vi "SLL DE AO Circular Buffer.vi"(6 "Pointers":T3=enum."Pointer 4", 7 "Options":T4=enum."Write N", 8 "error in (no error)":errorcluster, 11 "AO value Array":dbl[][](array[numeric])) -> (0 "error Out":errorcluster, 1 "Data Overflow?":T2, 2 "Output points":sgl[](array[numeric]), 3 "Output Data":sgl[][](array[numeric]))   [LabVIEW 2013]
doc: "This vi acts as a circular buffer for Analog input channel data storage. \nOutput Array- Column coresponds to single channel data.\nSingle Point data of all channels will avilable, When 'Data Point' case will executes.\nYou can get continous data in two mode 'Read Pointer 1' and 'Read Pointer 2'.\nInitializing Pointer is recommeded to avoid overflow\n\nCreated by Yogesh Redemptor, \nCopyright © 2009, Soliton Technologies.\nAll rights reserved."
uses:
  Controls/SLL DE AO Circular Buffer Options.ctl
  Controls/SLL DE Circular Buffer Pointers List.ctl
  Controls/SLL DE Circular Buffer Overflow Info.ctl
  Controls/SLL DE List of Analog Outputs.ctl
  Controls/SLL DE DAQ Parameters LV2Global Options.ctl
panel:
  in  "AO Channel Name Array":T1[](array[typedef])
  in  "AO value":dbl[](array[numeric])
  in  "AO Channel Name":T1
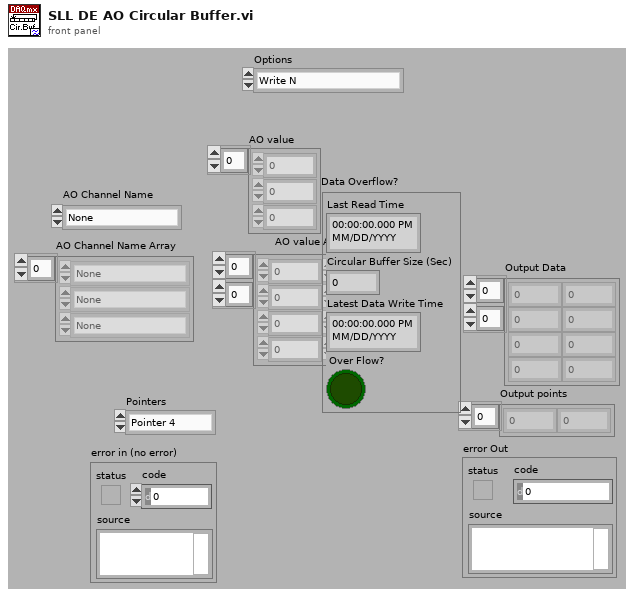
[diagram p1: front panel]
types:
  T1 = typedef "SLL DE List of Analog Outputs.ctl" = enum16{"None"}
  T2 = typedef "SLL DE Circular Buffer Overflow Info.ctl" = cluster{"Last Read Time":timestamp, "Circular Buffer Size (Sec)":dbl, "Latest Data Write Time":timestamp, "Over Flow?":bool}
  T3 = typedef "SLL DE Circular Buffer Pointers List.ctl" = enum16{"Graph Pointer", "File Log Pointer", "Pointer 3", "Pointer 4"}
  T4 = typedef "SLL DE AO Circular Buffer Options.ctl" = enum16{"Initialize", "Write 1", "Write N", "Read 1", "Read N", "Clear Data"}
  T5 = typedef "SLL DE DAQ Parameters LV2Global Options.ctl" = enum16{"Read", "Write"}
  T6 = cluster{"Buffer Length":i32, "Write Pointer":i32, "Write Time":timestamp, "AI Sampling Rate (Samples/Sec)":i32, "# Samples to write":i32}
  T7 = cluster{"Read Pointer X Pointer":i32, "Pointer X Overflow?":bool, "Read Pointer X Time":timestamp}
  T8 = typedef "SLL DE DAQ Engine Parameters.ctl" = cluster{"Enable Engines":cluster{"AI Enable":bool, "AO Enable":bool, "DI Enable":bool, "DO Enable":bool}, "DAQ Control Type":cluster{"Analog Input":enum16{"Finite", "Continuous", "Driver"}, "Analog Output":enum16{"Finite", "Continuous", "Driver"}, "Digital Input":enum16{"Finite", "Continuous", "Driver"}, "Digital Output":enum16{"Finite", "Continuous", "Driver"}}, "DAQ Parameters":cluster{"AI Sampling Rate (Samples/Sec)":dbl, "MvgAVG Window Size (# of Points)":i32, "Enable Filter":bool, "Enable MvgAVG":bool, "Circular Buffer Size (Sec)":dbl, "AO Sampling Rate (Samples/Sec)":dbl, "Graph Update Rate (Samples/Sec)":dbl, "File Logging Rate (Samples/Sec)":i32}, "AO Safe Values":cluster{"Analog Outputs Name":T1, "Analog Outputs Safe Value":dbl}[], "DO Safe Values":cluster{"Digital Outputs Name":T9, "Digital Outputs Safe Value":bool}[], "DO Interconnected Lines":cluster{"First DO Line":string, "Second DO Line":string}[], "AI Channels Unit":cluster{"Channel Name":T10, "Channel Type":T11}[], "Units Information":cluster{"Channel Type":T11, "Unit Text":string, "Maximum":dbl, "Minmum":dbl, "Increments":dbl}[]}
  T9 = typedef "SLL DE List of Digital Outputs.ctl" = enum16{"STATION1_START TEST", "STATION1_STOP TEST", "STATION1_LIGHT1", "STATION1_LIGHT2", "STATION1_LIGHT3", "STATION2_START TEST", "STATION2_STOP TEST", "STATION2_LIGHT1", "STATION2_LIGHT2", "STATION2_LIGHT3", "STATION3_START TEST", "STATION3_STOP TEST", "STATION3_LIGHT1", "STATION3_LIGHT2", "STATION3_LIGHT3", "STATION4_START TEST", "STATION4_STOP TEST", "STATION4_LIGHT1", "STATION4_LIGHT2", "STATION4_LIGHT3"}
  T10 = typedef "SLL DE List of Analog Inputs.ctl" = enum16{"None"}
  T11 = typedef "SLL DE List of AI Channel Type.ctl" = enum16{"Pressure", "Flow", "Temperature", "Time Scale", "Voltage", "Current", "Frequency", "Sound", "Speed", "Torque", "Distance", "Channel Type 1", "Channel Type 2", "Channel Type 3"}
  T12 = cluster{"Read Pointer X Pointer":i32, "Pointer X Overflow?":bool, "Read Pointer X Time":timestamp}[]
  T13 = cluster{"Read Pointer X Time":timestamp, "Circular Buffer Size (Sec)":dbl, "Write Time":timestamp, bool}
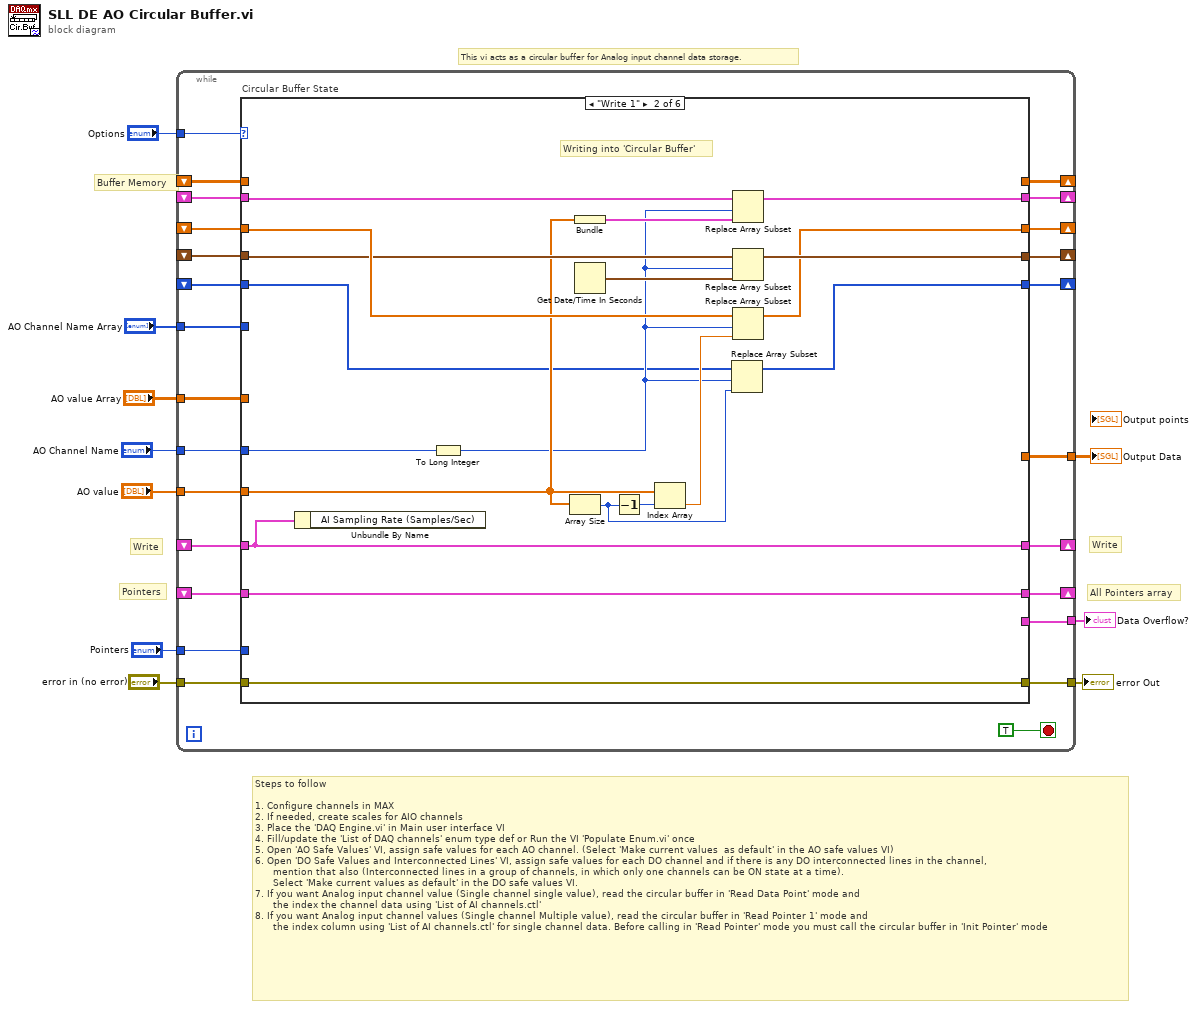
[diagram p0: block diagram]
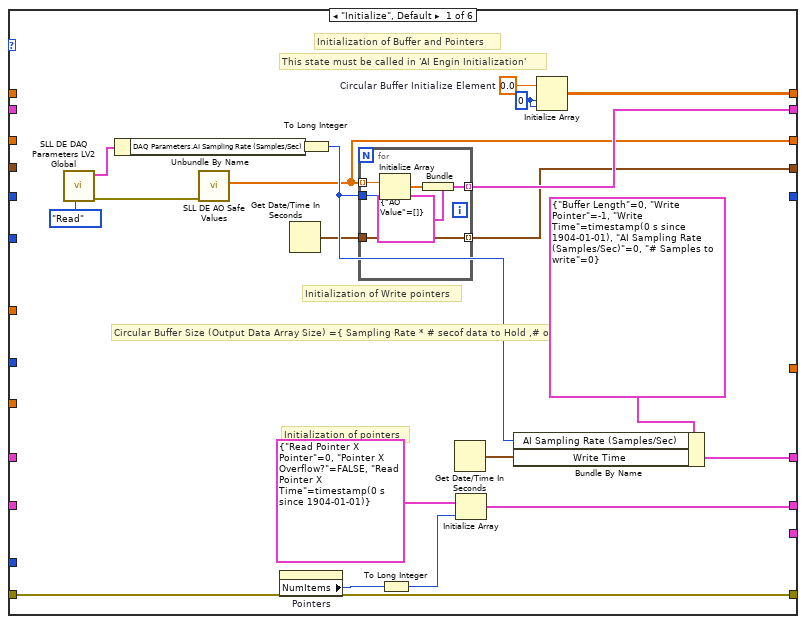
[diagram p2: hidden frame]
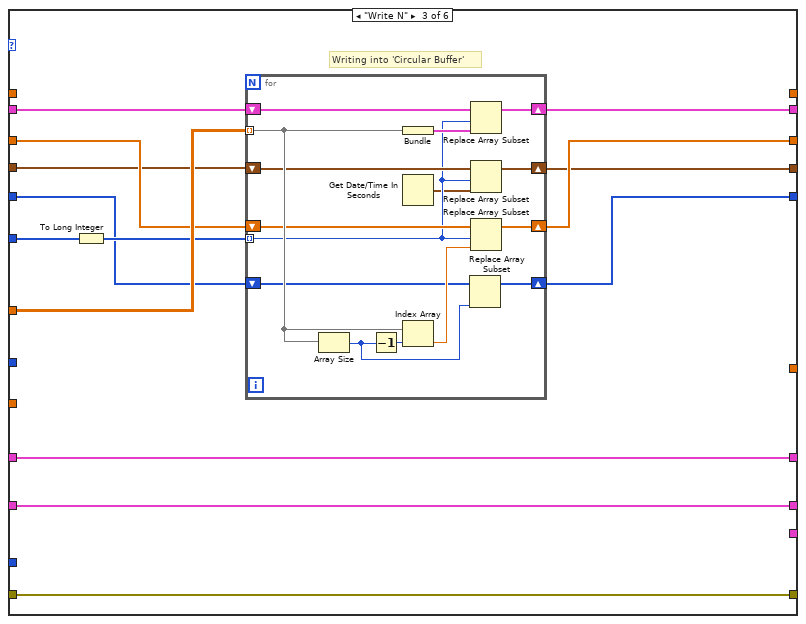
[diagram p3: hidden frame]
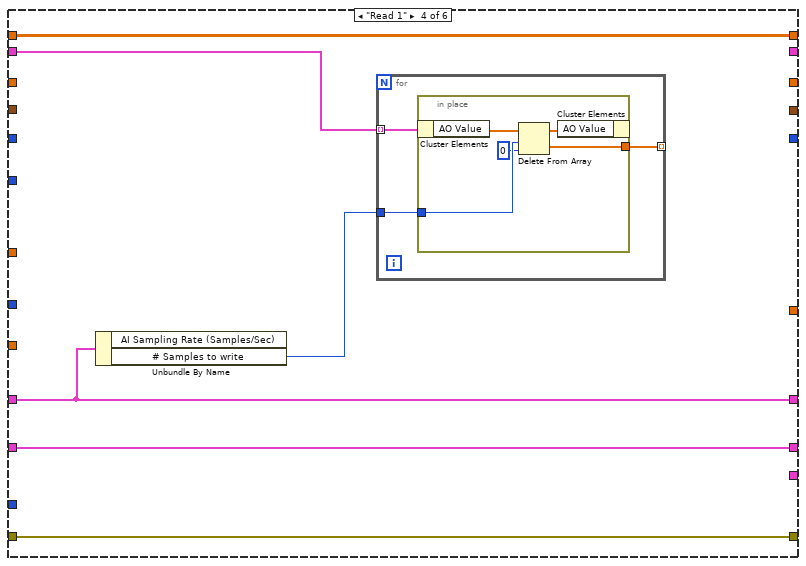
[diagram p4: hidden frame]
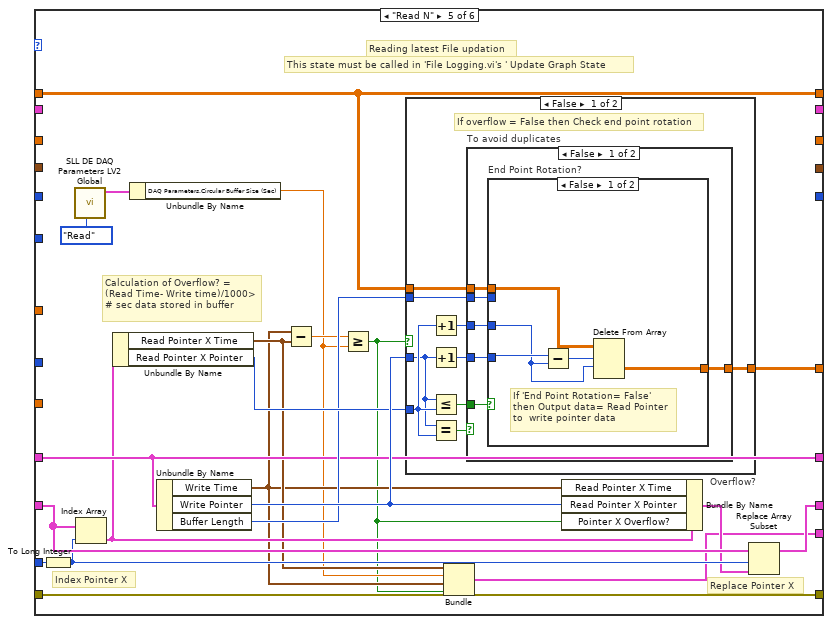
[diagram p5: hidden frame]
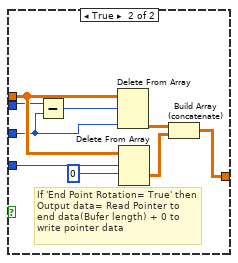
[diagram p6: hidden frame]
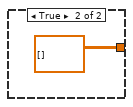
[diagram p7: hidden frame]
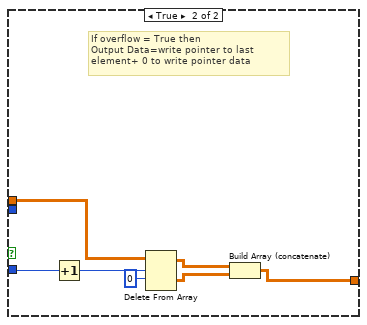
[diagram p8: hidden frame]
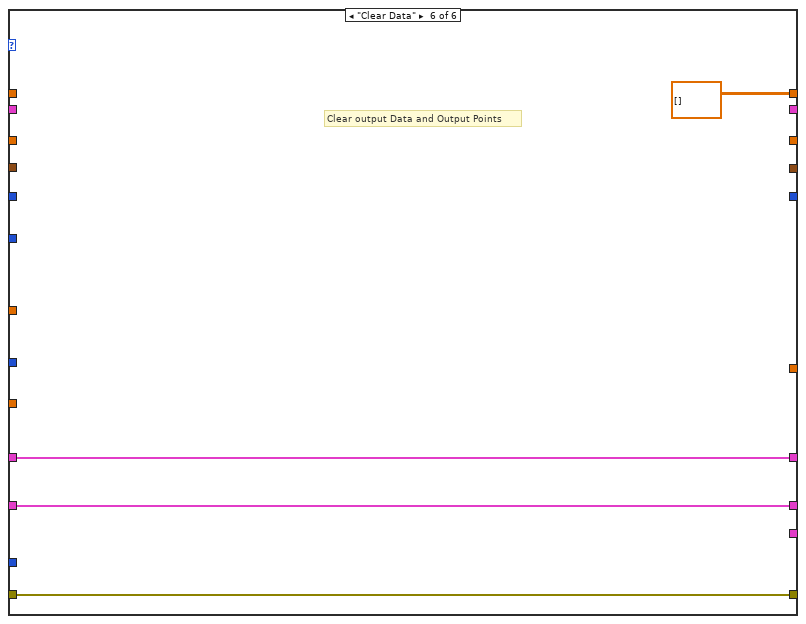
[diagram p9: hidden frame]
diagram:
  # "Steps to follow\n\n1.\tConfigure channels in MAX\n2.\tIf needed, create scales for AIO channels\n3.\tPlace the 'DAQ Engine.vi' in Main user interface VI\n4.\tFill/update the 'List of DAQ channels' enum type def or Run the VI 'Populate Enum.vi' once\n5.\tOpen 'AO Safe Values' VI, assign safe values for each AO channel. (Select 'Make current values  as default' in the AO safe values VI)\n6.\tOpen 'DO Safe Values and Interconnected Lines' VI, assign safe values for each DO channel and if there is any DO interconnected lines in the channel,\n      mention that also (Interconnected lines in a group of channels, in which only one channels can be ON state at a time). \n      Select 'Make current values as default' in the DO safe values VI.\n7.\tIf you want Analog input channel value (Single channel single value), read the circular buffer in 'Read Data Point' mode and \n      the index the channel data using 'List of AI channels.ctl' \n8.\tIf you want Analog input channel values (Single channel Multiple value), read the circular buffer in 'Read Pointer 1' mode and \n      the index column using 'List of AI channels.ctl' for single channel data. Before calling in 'Read Pointer' mode you must call the circular buffer in 'Init Pointer' mode"
  # "Buffer Memory"
  # "Write"
  # "Write"
  # "Pointers"
  # "All Pointers array"
  # "This vi acts as a circular buffer for Analog input channel data storage."
  n1 = while {
    tunnel: "Options" -> [w35]
    shift-right: [w33] -> _
    shift-left: _ -> [w31]
    shift-right: [w32] -> _
    shift-left: _ -> [w30]
    tunnel: "AO value Array" -> [w29]
    shift-right: [w28] -> _
    shift-left: _ -> [w27]
    tunnel: [w26] -> w9
    tunnel: "error in (no error)" -> [w25]
    tunnel: [w24] -> w7
    tunnel: "Pointers" -> [w23]
    tunnel: [w22] -> w4
    shift-right: [w21] -> _
    shift-left: _ -> [w20]
    tunnel: "AO Channel Name" -> [w19]
    tunnel: "AO value" -> [w18]
    tunnel: "AO Channel Name Array" -> [w17]
    shift-right: [w16] -> _
    shift-left: _ -> [w15]
    shift-right: [w14] -> _
    shift-left: _ -> [w13]
    shift-right: [w12] -> _
    shift-left: _ -> [w11]
    stop <- TRUE stop-if-true
    n2 = case "Circular Buffer State" shown="\"Write 1\"" w35 {
      tunnel: [w55 _ _ w114 w144 sgl[][] []] -> w33
      tunnel: [w51 w76 w94 w115 w133 w185] -> w32
      tunnel: w31 -> [_ _ _ w114 w144 _]
      tunnel: w30 -> [_ w76 w94 w115 w136 w185]
      tunnel: w29 -> [_ _ w92 _ _ _]
      tunnel: [w52 w75 w83 w112 w139 w184] -> w28
      tunnel: w27 -> [_ w75 w83 w112 w139 w184]
      tunnel: [_ _ _ _ w143 _] -> w26
      tunnel: w25 -> [w47 w80 w93 w113 w138 w182]
      tunnel: [w47 w80 w93 w113 w138 w182] -> w24
      tunnel: w23 -> [_ _ _ _ w137 _]
      tunnel: [_ _ _ _ w124 _] -> w22
      tunnel: [w41 w72 w88 _ _ _] -> w21
      tunnel: w20 -> [_ w79 w91 w111 _ _]
      tunnel: w19 -> [_ w67 _ _ _ _]
      tunnel: w18 -> [_ w66 _ _ _ _]
      tunnel: w17 -> [_ _ w90 _ _ _]
      tunnel: [w38 w73 w87 _ _ _] -> w16
      tunnel: w15 -> [_ w78 w86 _ _ _]
      tunnel: [w36 w74 w84 _ _ _] -> w14
      tunnel: w13 -> [_ w77 w85 _ _ _]
      tunnel: [_ w63 w81 _ _ _] -> w12
      tunnel: w11 -> [_ w62 w82 _ _ _]
      frame "Initialize", Default {
        w54 = sgl 0.0  # Circular Buffer Initialize Element
        w43 = 0 ("dimension size")
        # "Initialization of pointers"
        # "Initialization of Write pointers"
        # "This state must be called in 'AI Engin Initialization'"
        # "Initialization of Buffer and Pointers"
        # "Circular Buffer Size (Output Data Array Size) ={ Sampling Rate * # secof data to Hold ,# of AI Channels}"
        n3 = call "SLL DE DAQ Parameters LV2 Global.vi"("Option"=SLL_DE_DAQ_Parameters_LV2Global_Options."Read") -> ("Error out"=w40:errorcluster, "Global Info"=w48:T8)  [unwired: 9 in]
        n4 = Unbundle By Name(w48) -> ("DAQ Parameters.AI Sampling Rate (Samples/Sec)"=w42:dbl)
        n5 = call "SLL DE AO Safe Values.vi"("error in (no error)"=w40) -> ("AO Safe Values"=w38:dbl[])  [unwired: 8 in, 2 out]
        n6 = property on="Pointers" class="Enum (strict)"() -> ("NumItems"=w46:u32)  [unwired: 2 in, 2 out]
        n7 = Get Date/Time In Seconds() -> (seconds since 1Jan1904=w37:timestamp)
        n8 = To Long Integer(number=w42) -> (32bit integer=w39:i32)
        n9 = for {
          tunnel: w38 -> [w61] mode=indexing
          tunnel: w39 -> [w60]
          tunnel: [w58] -> w41 mode=indexing
          tunnel: w37 -> [w57]
          tunnel: [w57] -> w36 mode=indexing
          n10 = Initialize Array(w61, w60) -> (w59:dbl[])
          n11 = Bundle(cluster=cluster{"AO Value":dbl[]} {"AO Value"=[]}, "AO Value"=w59) -> (w58:cluster{"AO Value":dbl[]})
        }
        n12 = To Long Integer(number=w46) -> (32bit integer=w45:i32)
        n13 = Get Date/Time In Seconds() -> (seconds since 1Jan1904=w44:timestamp)
        n14 = Initialize Array(T7 {"Read Pointer X Pointer"=0, "Pointer X Overflow?"=FALSE, "Read Pointer X Time"=timestamp(0 s since 1904-01-01)} ("Graph"), w45) -> (w51:T12)
        n15 = Bundle By Name(cluster=T6 {"Buffer Length"=0, "Write Pointer"=-1, "Write Time"=timestamp(0 s since 1904-01-01), "AI Sampling Rate (Samples/Sec)"=0, "# Samples to write"=0} ("Cluster"), "AI Sampling Rate (Samples/Sec)"=w39, "Write Time"=w44) -> (w52:T6)
        n16 = Initialize Array(w54, w43, w43) -> (w55:sgl[][])
      }
      frame "Write 1" {
        # "Writing into 'Circular Buffer'"
        n17 = Unbundle By Name(w75) -> ()  [unwired: 1 out]
        n18 = To Long Integer(number=w67) -> (32bit integer=w64:i32)
        n19 = Array Size(array=w66) -> (size(s)=w65:i32)
        n20 = Bundle("AO value"=w66) -> (w71:cluster{"AO value":dbl[]})  [unwired: 1 in]
        n21 = Get Date/Time In Seconds() -> (seconds since 1Jan1904=w68:timestamp)
        n22 = Decrement(x=w65) -> (x-1=w70:i32)
        n23 = Index Array(array=w66, index=w70) -> (element=w69:dbl)
        n24 = Replace Array Subset(array=w62, new element=w65, index=w64) -> (w63:i32[])
        n25 = Replace Array Subset(array=w79, new element=w71, index=w64) -> (w72:cluster{"AO Value":dbl[]}[])
        n26 = Replace Array Subset(array=w77, new element=w68, index=w64) -> (w74:timestamp[])
        n27 = Replace Array Subset(array=w78, new element=w69, index=w64) -> (w73:dbl[])
      }
      frame "Write N" {
        # "Writing into 'Circular Buffer'"
        n28 = To Long Integer(number=w90) -> (32bit integer=w89:i32[])
        n29 = for {
          tunnel: w92 -> [w105] mode=indexing
          shift-right: [w108] -> w88
          shift-left: w91 -> [w109]
          tunnel: w89 -> [w99] mode=indexing
          shift-right: [w103] -> w87
          shift-left: w86 -> [w102]
          shift-right: [w100] -> w84
          shift-left: w85 -> [w101]
          shift-right: [w96] -> w81
          shift-left: w82 -> [w95]
          n30 = Array Size(array=w105) -> (size(s)=w97:i32)
          n31 = Decrement(x=w97) -> (x-1=w106:i32)
          n32 = Bundle("AO value Array"=w105) -> (w107:cluster{"AO value Array":dbl[]})  [unwired: 1 in]
          n33 = Get Date/Time In Seconds() -> (seconds since 1Jan1904=w98:timestamp)
          n34 = Index Array(array=w105, index=w106) -> (element=w104:dbl)
          n35 = Replace Array Subset(array=w95, new element=w97) -> (w96:i32[])  [unwired: 1 in]
          n36 = Replace Array Subset(array=w109, new element=w107, index=w99) -> (w108:cluster{"AO Value":dbl[]}[])
          n37 = Replace Array Subset(array=w101, new element=w98, index=w99) -> (w100:timestamp[])
          n38 = Replace Array Subset(array=w102, new element=w104, index=w99) -> (w103:dbl[])
        }
      }
      frame "Read 1" {
        n39 = Unbundle By Name(w112) -> ("# Samples to write"=w110:i32)  [unwired: 1 out]
        n40 = for {
          tunnel: w111 -> [w118] mode=indexing
          tunnel: w110 -> [w117]
          tunnel: [w116] -> _ mode=indexing
          n41 = in-place {
            in-place-border: w117 -> [w120]
            in-place-border: [w121] -> w116
            n42 = in-place-cluster #1(w118) -> ("AO Value"=w123:dbl[])
            n43 = Delete From Array(array=w123, length=w120, index=0) -> (deleted portion=w121:dbl[], array with subset deleted=w122:dbl[])
            n44 = in-place-cluster #1("AO Value"=w122) -> ()  [unwired: 1 out]
          }
        }
      }
      frame "Read N" {
        # "Replace Pointer X"
        # "Index Pointer X"
        # "Calculation of Overflow? = \n(Read Time- Write time)/1000> # sec data stored in buffer"
        # "Reading latest File updation"
        # "This state must be called in 'File Logging.vi's ' Update Graph State"
        n45 = To Long Integer(number=w137) -> (32bit integer=w135:i32)
        n46 = call "SLL DE DAQ Parameters LV2 Global.vi"("Option"=SLL_DE_DAQ_Parameters_LV2Global_Options."Read") -> ("Global Info"=w131:T8)  [unwired: 9 in, 1 out]
        n47 = Index Array(array=w136, index=w135) -> (element=w132:T7)
        n48 = Unbundle By Name(w132) -> ("Read Pointer X Time"=w128:timestamp, "Read Pointer X Pointer"=w141:i32)
        n49 = Unbundle By Name(w131) -> ("DAQ Parameters.Circular Buffer Size (Sec)"=w126:dbl)
        n50 = Unbundle By Name(w139) -> ("Write Time"=w127:timestamp, "Write Pointer"=w142:i32, "Buffer Length"=w140:i32)
        n51 = Subtract(x=w127, y=w128) -> (x-y=w129:dbl)
        n52 = Greater Or Equal?(x=w129, y=w126) -> (x >= y?=w125:bool)
        n53 = case "Overflow?" shown="False" w125 {
          tunnel: w144 -> [w152 w179]
          tunnel: [w151 w177] -> w143
          tunnel: w142 -> [w147 w181]
          tunnel: w141 -> [w148 _]
          tunnel: w140 -> [w150 _]
          frame False {
            # "If overflow = False then Check end point rotation"
            n54 = Increment(x=w148) -> (x+1=w145:i32)
            n55 = Increment(x=w147) -> (x+1=w146:i32)
            n56 = Less Or Equal?(x=w147, y=w148) -> (x <= y?=w153:bool)
            n57 = Equal?(x=w147, y=w148) -> (x = y?=w149:bool)
            n58 = case "To avoid duplicates" shown="False" w149 {
              tunnel: w153 -> [w159 _]
              tunnel: w152 -> [w158 _]
              tunnel: [w157 sgl[][] []] -> w151
              tunnel: w150 -> [w156 _]
              tunnel: w145 -> [w155 _]
              tunnel: w146 -> [w154 _]
              frame False {
                n59 = case "End Point Rotation?" shown="False" w159 {
                  tunnel: w158 -> [w164 w173]
                  tunnel: [w163 w170] -> w157
                  tunnel: w155 -> [w160 w167]
                  tunnel: w154 -> [w162 w166]
                  tunnel: w156 -> [_ w169]
                  frame False {
                    # "If 'End Point Rotation= False' then Output data= Read Pointer to  write pointer data"
                    n60 = Subtract(x=w162, y=w160) -> (x-y=w161:i32)
                    n61 = Delete From Array(array=w164, length=w161, index (row)=w160) -> (deleted portion=w163:sgl[][])  [unwired: 1 in, 1 out]
                  }
                  frame True {
                    # "If 'End Point Rotation= True' then Output data= Read Pointer to end data(Bufer length) + 0 to write pointer data"
                    n62 = Subtract(x=w169, y=w167) -> (x-y=w168:i32)
                    n63 = Delete From Array(array=w173, length=w168, index (row)=w167) -> (deleted portion=w172:sgl[][])  [unwired: 1 in, 1 out]
                    n64 = Delete From Array(array=w173, length=w166, index (row)=0) -> (deleted portion=w171:sgl[][])  [unwired: 1 in, 1 out]
                    n65 = Build Array (concatenate)(w172, w171) -> (w170:sgl[][])
                  }
                }
              }
              frame True {
              }
            }
          }
          frame True {
            # "If overflow = True then\nOutput Data=write pointer to last element+ 0 to write pointer data"
            n66 = Increment(x=w181) -> (x+1=w175:i32)
            n67 = Delete From Array(array=w179, length=w175, index (row)=0) -> (deleted portion=w178:sgl[][], array with subset deleted=w176:sgl[][])  [unwired: 1 in]
            n68 = Build Array (concatenate)(w176, w178) -> (w177:sgl[][])
          }
        }
        n69 = Bundle("Read Pointer X Time"=w128, "Circular Buffer Size (Sec)"=w126, "Write Time"=w127, w125) -> (w124:T13)  [unwired: 1 in]
        n70 = Bundle By Name(cluster=w132, "Read Pointer X Time"=w127, "Read Pointer X Pointer"=w142, "Pointer X Overflow?"=w125) -> (w134:T7)
        n71 = Replace Array Subset(array=w136, new element=w134, index=w135) -> (w133:T12)
      }
      frame "Clear Data" {
        # "Clear output Data and Output Points"
      }
    }
  }
  "Output Data" <- w9
  "error Out" <- w7
  "Data Overflow?" <- w4
